vi "stream_data.vi"(5 "DATA STREAMING":bool=TRUE, 11 "error in (no error)":errorcluster) -> (15 "error out":errorcluster)   [LabVIEW 2017, in "ZBOX_IS.lvlib"]
uses:
  ZBOX_IS.lvlib
panel:
  out "HI to LO":bool
  out "LO to HI":bool
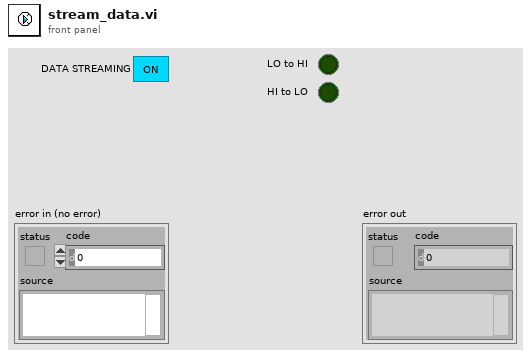
[diagram p1: front panel]
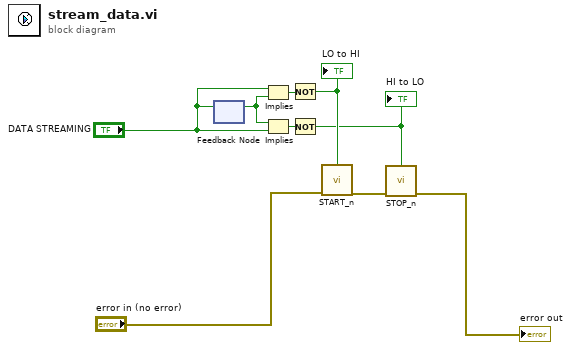
[diagram p0: block diagram]
diagram:
  n1 = feedback #1() -> (w8:bool)  [unwired: 1 out]
  n2 = feedback-in #1("DATA STREAMING") -> ()
  n3 = Implies(1:w8, 2:"DATA STREAMING") -> (0:w6:bool)
  n4 = Implies(1:"DATA STREAMING", 2:w8) -> (0:w7:bool)
  n5 = Not(x=w6) -> (.not. x?=w5:bool)
  "LO to HI" <- w5
  n6 = Not(x=w7) -> (.not. x?=w1:bool)
  "HI to LO" <- w1
  n7 = call "START_n.vi"("execute"=w5, "error in (no error)"="error in (no error)") -> ("error out"=w9:errorcluster)  [unwired: 12 in, 1 out]
  n8 = call "STOP_n.vi"("execute"=w1, "error in (no error)"=w9) -> ("error out"=→"error out":errorcluster)  [unwired: 12 in, 1 out]
